vi "ADDR to DevAddr.vi"(1 "ADDR pin":bool) -> (0 "Slave Address (7-bit)":u8)   [LabVIEW 2021]
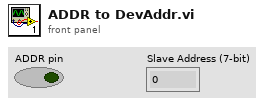
[diagram p1: front panel]
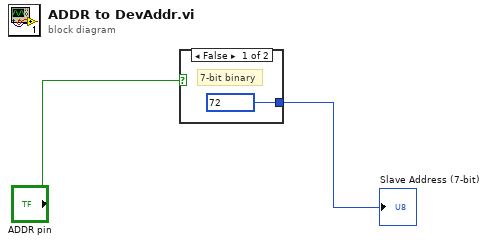
[diagram p0: block diagram]
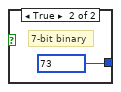
[diagram p2: hidden frame]
diagram:
  n1 = case shown="False" "ADDR pin" {
    tunnel: [u8 72 ("Slave Address (7-bit)") u8 73 ("Slave Address (7-bit)")] -> w1
    frame False {
      # "7-bit binary"
    }
    frame True {
      # "7-bit binary"
    }
  }
  "Slave Address (7-bit)" <- w1
